vi "RandomGennerateI32.vi"(10 "limit":dbl=40.0 format="%#_13g") -> (3 "32位整型":i32)   [LabVIEW 2018, in "RandomMoveBool.lvclass"]
uses:
  RandomMoveBool.lvclass
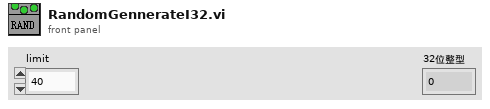
[diagram p1: front panel]
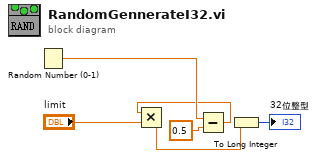
[diagram p0: block diagram]
diagram:
  n1 = Random Number (0-1)() -> (number: 0 to 1=w3:dbl)
  n2 = Subtract(x=w3, y=0.5) -> (x-y=w2:dbl)
  n3 = Multiply(x=w2, y="limit") -> (x*y=w1:dbl)
  n4 = To Long Integer(number=w1) -> (32bit integer=→"32位整型":i32)
